vi "UpdateFullImage.vi"(0 "Display Settings":T1={"Show MCS"=TRUE, "Show Image"=TRUE, "Color coding"=0, "Plane"=0, "Threshold"={"max"=1000, "min"=1000}} {"Color coding" items=["Color Gradient", "False Color"]}) -> ()   [LabVIEW 2009]
uses:
  DisplaySettings.ctt
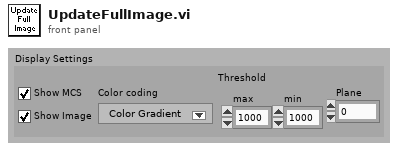
[diagram p1: front panel]
types:
  T1 = typedef "DisplaySettings.ctt" = cluster{"Show MCS":bool, "Show Image":bool, "Color coding":u16, "Plane":u32, "Threshold":cluster{"max":u32, "min":u32}}
  T2 = typedef "ScannedImage.ctl" = cluster{"BinningMicroS":dbl, "OverflowConstant":dbl, "MacrotimeCycle":dbl, "Trace":u32[][][][], "Retrace":u32[][][][], "current line":i32, "current plane":i32}
  T3 = typedef "DAQLinescanVisualization.ctt" = cluster{"Threshold":u32, "Trace Window #":u32, "IMAQ Trace":T4, "Retrace Window #":u32, "IMAQ Retrace":T4}
  T4 = typedef "IMAQ Image.ctl" = refnum<image>
  T5 = typedef "ImageSettings.ctt" = cluster{"Start Position (µm)":cluster{"x":dbl, "y":dbl, "z":dbl}, "End Position (µm)":cluster{"x":dbl, "y":dbl, "z":dbl}, "Image Resolution (nm/pixel)":cluster{"x":dbl, "y":dbl, "z":dbl}, "Image Size (µm)":cluster{"x":dbl, "y":dbl, "z":dbl}, "Image Size (pixel)":cluster{"x":u32, "y":u32, "z":u32}, "Time Resolution\n(ms/pixel)":dbl, "1st Axis":u16, "2nd Axis":u16, "Retrace":bool, "Estimated Time":string}
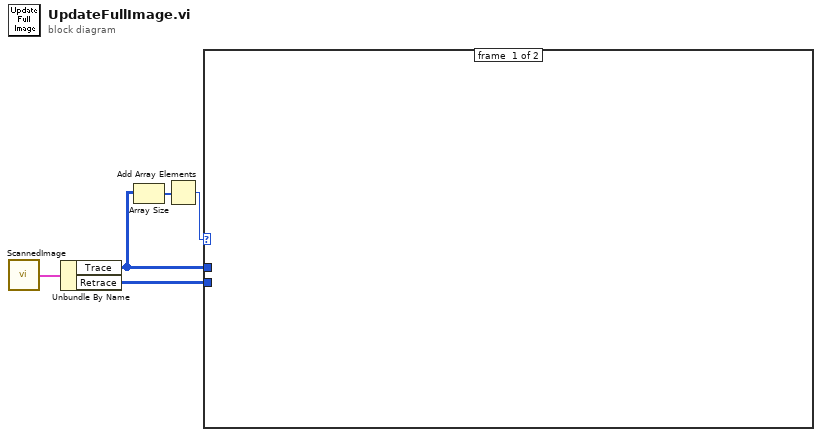
[diagram p0: block diagram]
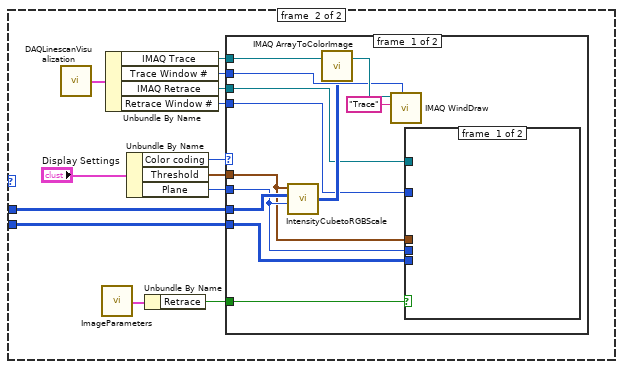
[diagram p2: hidden frame]
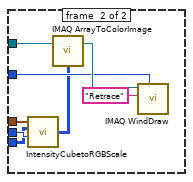
[diagram p3: hidden frame]
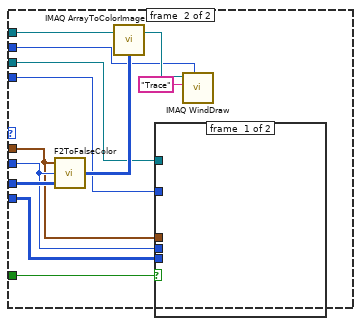
[diagram p4: hidden frame]
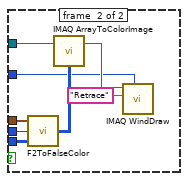
[diagram p5: hidden frame]
diagram:
  n1 = call "ScannedImage.vi"() -> ("Scanned Image (output)"=w4:T2)  [unwired: 2 in]
  n2 = Unbundle By Name(w4) -> ("Trace"=w3:u32[][][][], "Retrace"=w5:u32[][][][])
  n3 = Array Size(array=w3) -> (size(s)=w2:i32[])
  n4 = Add Array Elements(numeric array=w2) -> (sum=w1:i32)
  n5 = case shown="1, Default" w1 {
    tunnel: w5 -> [_ w11]
    tunnel: w3 -> [_ w6]
    frame #0 {
    }
    frame #1 {
      n6 = call "DAQLinescanVisualization.vi"() -> ("Visualization (output)"=w14:T3)  [unwired: 2 in]
      n7 = call "ImageParameters.vi"() -> ("Image Parameters (output)"=w12:T5)  [unwired: 2 in]
      n8 = Unbundle By Name(w14) -> ("IMAQ Trace"=w15:T4, "Trace Window #"=w16:u32, "IMAQ Retrace"=w18:T4, "Retrace Window #"=w17:u32)
      n9 = Unbundle By Name("Display Settings") -> ("Color coding"=w10:u16, "Threshold"=w9:cluster{"max":u32, "min":u32}, "Plane"=w8:u32)
      n10 = Unbundle By Name(w12) -> ("Retrace"=w13:bool)
      n11 = case shown="1" w10 {
        tunnel: w6 -> [w30 w50]
        tunnel: w8 -> [w28 w49]
        tunnel: w9 -> [w19 w39]
        tunnel: w13 -> [w29 w47]
        tunnel: w11 -> [w27 w48]
        tunnel: w15 -> [w24 w45]
        tunnel: w16 -> [w23 w42]
        tunnel: w17 -> [w21 w41]
        tunnel: w18 -> [w20 w40]
        frame #0 {
          n12 = call "IntensityCubetoRGBScale.vi"("Plane"=w28, "Trace"=w30, "threshold"=w19) -> ("RGB Scale"=w22:u32[][])  [unwired: 1 in]
          n13 = call "IMAQ ArrayToColorImage"("Image Pixels (U32)"=w22, "Image"=w24) -> ("Image Out"=w25:T4)  [unwired: 3 in, 1 out]
          n14 = call "IMAQ WindDraw"("Window Number (0...15)"=w23, "Title"="Trace", "Image"=w25) -> ()  [unwired: 7 in, 2 out]
          n15 = case shown="True" w29 {
            tunnel: w28 -> [_ w38]
            tunnel: w27 -> [_ w37]
            tunnel: w21 -> [_ w34]
            tunnel: w20 -> [_ w33]
            tunnel: w19 -> [_ w31]
            frame #0 {
            }
            frame #1 {
              n16 = call "IntensityCubetoRGBScale.vi"("Plane"=w38, "Trace"=w37, "threshold"=w31) -> ("RGB Scale"=w32:u32[][])  [unwired: 1 in]
              n17 = call "IMAQ ArrayToColorImage"("Image Pixels (U32)"=w32, "Image"=w33) -> ("Image Out"=w36:T4)  [unwired: 3 in, 1 out]
              n18 = call "IMAQ WindDraw"("Window Number (0...15)"=w34, "Title"="Retrace", "Image"=w36) -> ()  [unwired: 7 in, 2 out]
            }
          }
        }
        frame #1 {
          n19 = call "F2ToFalseColor.vi"("Intensity"=w50, "Plane"=w49, "Threshold (max)"=w39) -> ("FalseColor"=w44:u32[][])
          n20 = call "IMAQ ArrayToColorImage"("Image Pixels (U32)"=w44, "Image"=w45) -> ("Image Out"=w43:T4)  [unwired: 3 in, 1 out]
          n21 = case shown="True" w47 {
            tunnel: w49 -> [_ w58]
            tunnel: w48 -> [_ w57]
            tunnel: w41 -> [_ w53]
            tunnel: w40 -> [_ w52]
            tunnel: w39 -> [_ w51]
            frame #0 {
            }
            frame #1 {
              n22 = call "F2ToFalseColor.vi"("Intensity"=w57, "Plane"=w58, "Threshold (max)"=w51) -> ("FalseColor"=w54:u32[][])
              n23 = call "IMAQ ArrayToColorImage"("Image Pixels (U32)"=w54, "Image"=w52) -> ("Image Out"=w56:T4)  [unwired: 3 in, 1 out]
              n24 = call "IMAQ WindDraw"("Window Number (0...15)"=w53, "Title"="Retrace", "Image"=w56) -> ()  [unwired: 7 in, 2 out]
            }
          }
          n25 = call "IMAQ WindDraw"("Window Number (0...15)"=w42, "Title"="Trace", "Image"=w43) -> ()  [unwired: 7 in, 2 out]
        }
      }
    }
  }
